vi "load configuration file.vi"(11 "Waveform chart":refnum<vi>) -> (2 "selected parameters":string[](array[string]), 3 "Waveform chart OUT":refnum<vi>)   [LabVIEW 2016]
uses:
  configuration file type def.ctl
  Communication Global variables.vi
  <vilib>/addons/_JKI.lib/Serialization/JSON/JKI JSON Serialization.lvlib
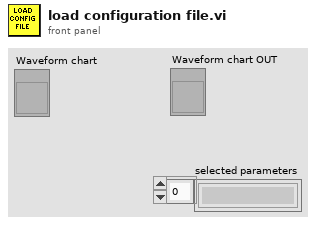
[diagram p1: front panel]
types:
  T1 = typedef "configuration file type def.ctl" = cluster{"selected parameters":string[], "REST URL":string, "UDP port":u16, "XScale.Minimum":dbl, "XScale.Maximum":dbl, "Yscale mins":dbl[], "Yscale maxs":dbl[], "Yscale colors":u32[], "LegNumRows":u32, "plot colors":u32[], "plot pointstyles":u8[], "plot names":string[], "plot yscale selections":u32[], "plot visibles":bool[]}
  T2 = enum16{"open", "replace", "create", "open or create", "replace or create", "replace or create with confirmation"}
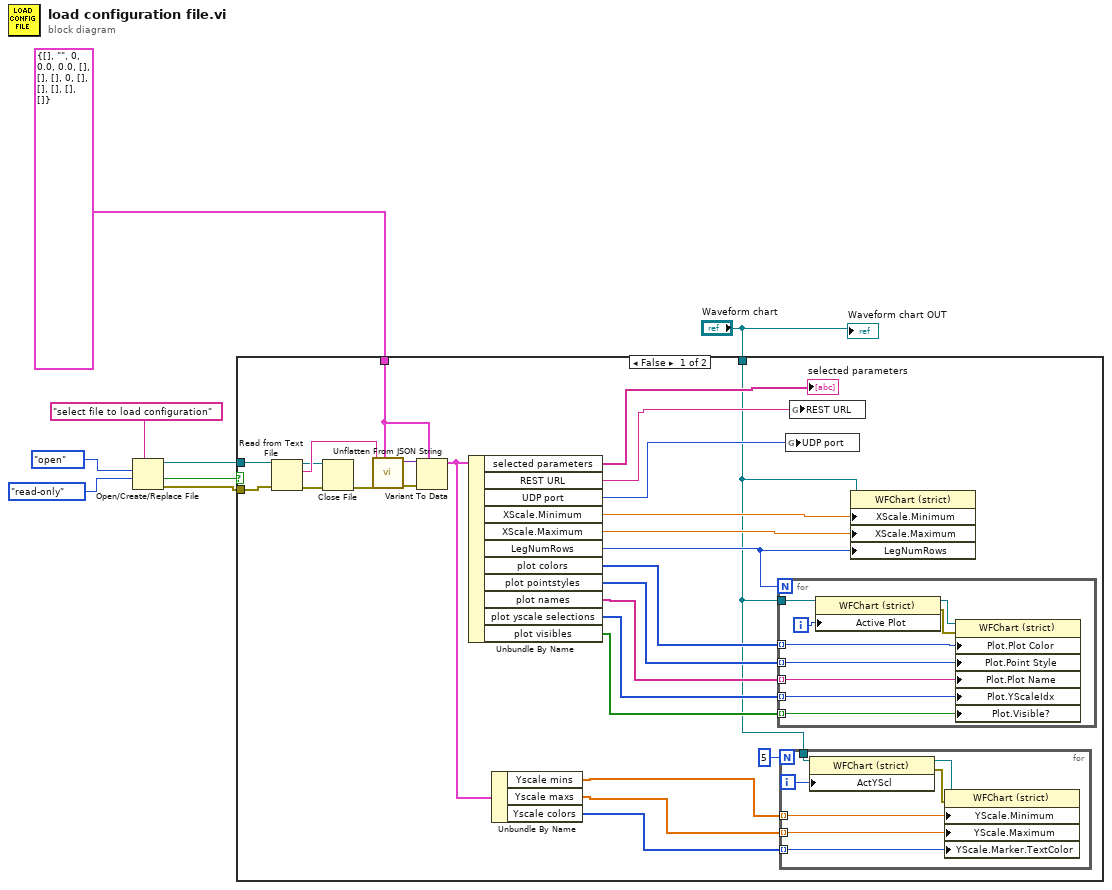
[diagram p0: block diagram]
diagram:
  n1 = Open/Create/Replace File(prompt="select file to load configuration", operation (0:open)=T2."open", access (0:read/write)=enum16{"read/write", "read-only", "write-only"}."read-only") -> (refnum out=w3:refnum<file>, cancelled=w7:bool, error out=w4:errorcluster)  [unwired: 3 in]
  n2 = case shown="False" w7 {
    tunnel: w4 -> [w34 _]
    tunnel: w3 -> [w33 _]
    tunnel: T1 {"selected parameters"=[], "REST URL"="", "UDP port"=0, "XScale.Minimum"=0.0, "XScale.Maximum"=0.0, "Yscale mins"=[], "Yscale maxs"=[], "Yscale colors"=[], "LegNumRows"=0, "plot colors"=[], "plot pointstyles"=[], "plot names"=[], "plot yscale selections"=[], "plot visibles"=[]} ("output cluster") -> [w28 _]
    tunnel: "Waveform chart" -> [w11 _]
    frame False {
      n3 = Read from Text File(file (use dialog)=w33, error in=w34) -> (refnum out=w9:refnum<file>, text=w32:string, error out=w31:errorcluster)  [unwired: 2 in, 1 out]
      n4 = Close File(refnum=w9, error in=w31) -> (error out=w10:errorcluster)  [unwired: 1 out]
      n5 = call <vilib>:"Unflatten From JSON String.vi"("Type and Defaults"=w28, "error in (no error)"=w10, "JSON String"=w32) -> ("error out"=w30:errorcluster, "Variant"=w29:variant)  [unwired: 7 in]
      n6 = Variant To Data(error in=w30, type=w28, Variant=w29) -> (data=w16:T1)  [unwired: 1 out]
      n7 = Unbundle By Name(w16) -> ("selected parameters"=→"selected parameters":string[], "REST URL"=w26:string, "UDP port"=w25:u16, "XScale.Minimum"=w24:dbl, "XScale.Maximum"=w23:dbl, "LegNumRows"=w22:u32, "plot colors"=w21:u32[], "plot pointstyles"=w20:u8[], "plot names"=w19:string[], "plot yscale selections"=w18:u32[], "plot visibles"=w17:bool[])
      n8 = Unbundle By Name(w16) -> ("Yscale mins"=w14:dbl[], "Yscale maxs"=w13:dbl[], "Yscale colors"=w12:u32[])
      n9 = for {
        N: w22 -> [_]
        tunnel: w11 -> [w49]
        tunnel: w21 -> [w46] mode=indexing
        tunnel: w20 -> [w45] mode=indexing
        tunnel: w19 -> [w44] mode=indexing
        tunnel: w18 -> [w43] mode=indexing
        tunnel: w17 -> [w42] mode=indexing
        i -> [w50]
        n10 = property class="WFChart (strict)"(reference=w49, "Active Plot"=w50) -> (reference out=w48:refnum<vi>, error out=w47:errorcluster)  [unwired: 1 in]
        n11 = property class="WFChart (strict)"(reference=w48, error in=w47, "Plot.Plot Color"=w46, "Plot.Point Style"=w45, "Plot.Plot Name"=w44, "Plot.YScaleIdx"=w43, "Plot.Visible?"=w42) -> ()  [unwired: 2 out]
      }
      n12 = for {
        N: 5 -> [_]
        tunnel: w14 -> [w38] mode=indexing
        tunnel: w13 -> [w37] mode=indexing
        tunnel: w12 -> [w36] mode=indexing
        tunnel: w11 -> [w35]
        i -> [w41]
        n13 = property class="WFChart (strict)"(reference=w35, "ActYScl"=w41) -> (reference out=w40:refnum<vi>, error out=w39:errorcluster)  [unwired: 1 in]
        n14 = property class="WFChart (strict)"(reference=w40, error in=w39, "YScale.Minimum"=w38, "YScale.Maximum"=w37, "YScale.Marker.TextColor"=w36) -> ()  [unwired: 2 out]
      }
      n15 = global write "Communication Global variables.vi" "UDP port"(w25) -> ()
      n16 = global write "Communication Global variables.vi" "REST URL"(w26) -> ()
      n17 = property class="WFChart (strict)"(reference=w11, "XScale.Minimum"=w24, "XScale.Maximum"=w23, "LegNumRows"=w22) -> ()  [unwired: 1 in, 2 out]
    }
    frame True {
      # "cancelled"
    }
  }
  "Waveform chart OUT" <- "Waveform chart"
